vi "Maxi Gauge-ConverIntIntEngEng.vi"(0 "String in":string, 1 "W/R [W: Int in; Str out ]":bool, 5 "Integer1 in":u8, 7 "Integer2 in":u8, 9 "Eng1 in":dbl format="%.2e", 11 "Eng2 in":dbl format="%.2e") -> (4 "String out":string, 6 "Integer1 out":u8, 8 "Integer2 out":u8, 10 "Eng1 out":dbl format="%.2e", 15 "Eng2 out":dbl format="%.2e")   [LabVIEW 2013, in "Maxi Gauge.lvlib"]
uses:
  <instrlib>/Maxi Gauge/Maxi Gauge.lvlib
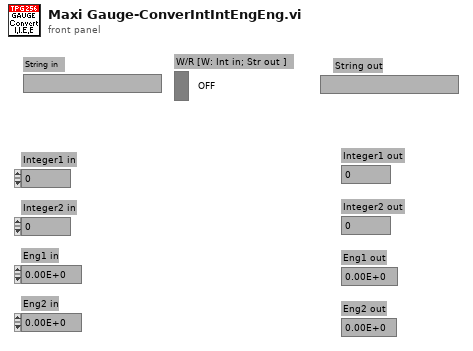
[diagram p1: front panel]
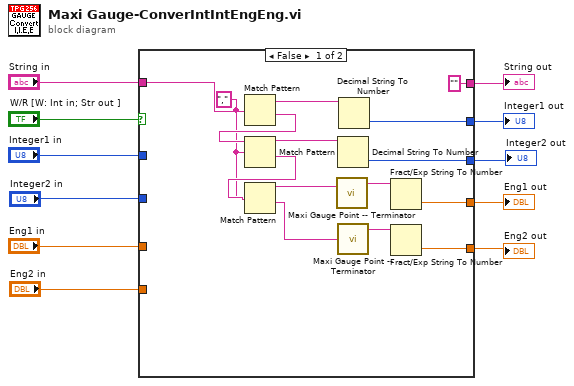
[diagram p0: block diagram]
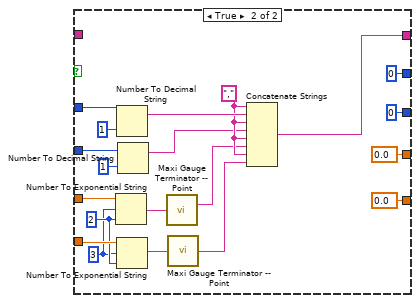
[diagram p2: hidden frame]
diagram:
  n1 = case shown="FALSE" "W/R [W: Int in; Str out ]" {
    tunnel: "Integer1 in" -> [_ w46]
    tunnel: "Eng1 in" -> [_ w45]
    tunnel: "Eng2 in" -> [_ w44]
    tunnel: ["" w40] -> w7
    tunnel: "String in" -> [w24 _]
    tunnel: [w23 0] -> w5
    tunnel: [w20 0.0] -> w4
    tunnel: [w19 0.0] -> w3
    tunnel: "Integer2 in" -> [_ w32]
    tunnel: [w17 0] -> w1
    frame False {
      w12 = "," ("regular expression")
      n2 = Match Pattern(string=w24, regular expression=w12) -> (before substring=w26:string, after substring=w25:string)  [unwired: 1 in, 2 out]
      n3 = Match Pattern(string=w25, regular expression=w12) -> (before substring=w13:string, after substring=w16:string)  [unwired: 1 in, 2 out]
      n4 = Match Pattern(string=w16, regular expression=w12) -> (before substring=w15:string, after substring=w14:string)  [unwired: 1 in, 2 out]
      n5 = call <instrlib>:"Maxi Gauge Point -- Terminator.vi"("Eingangstring"=w15) -> ("Ausgangstring"=w22:string)
      n6 = Decimal String To Number(string=w13) -> (number=w17:i32)  [unwired: 2 in, 1 out]
      n7 = call <instrlib>:"Maxi Gauge Point -- Terminator.vi"("Eingangstring"=w14) -> ("Ausgangstring"=w21:string)
      n8 = Decimal String To Number(string=w26) -> (number=w23:i32)  [unwired: 2 in, 1 out]
      n9 = Fract/Exp String To Number(string=w22) -> (number=w19:dbl)  [unwired: 3 in, 1 out]
      n10 = Fract/Exp String To Number(string=w21) -> (number=w20:dbl)  [unwired: 3 in, 1 out]
    }
    frame True {
      w34 = i16 3 ("width (-)")
      w35 = i16 2 ("width (-)")
      w31 = ","
      n11 = Number To Exponential String(number=w45, precision (6)=w35, 3:w34) -> (E-format string=w43:string)  [unwired: 1 in]
      n12 = Number To Decimal String(number=w46, width (-)=i16 1) -> (decimal integer string=w41:string)
      n13 = Number To Exponential String(number=w44, precision (6)=w35, 3:w34) -> (E-format string=w42:string)  [unwired: 1 in]
      n14 = Number To Decimal String(number=w32, width (-)=i16 1) -> (decimal integer string=w28:string)
      n15 = call <instrlib>:"Maxi Gauge Terminator -- Point.vi"("Eingangstring"=w43) -> ("Ausgangstring"=w30:string)
      n16 = call <instrlib>:"Maxi Gauge Terminator -- Point.vi"("Eingangstring"=w42) -> ("Ausgangstring"=w29:string)
      n17 = Concatenate Strings(w31, w41, w31, w28, w31, w30, w31, w29) -> (w40:string)
    }
  }
  "String out" <- w7
  "Integer1 out" <- w5
  "Eng1 out" <- w3
  "Eng2 out" <- w4
  "Integer2 out" <- w1
